vi "搜索变量函数.vi"(8 "错误输入":errorcluster caption="错误输入（无错误）", 11 "引用":refnum<k24>) -> (0 "错误输出":errorcluster, 1 "输出数组":string[](array[string]), 3 "引用输出":refnum<k24>)   [LabVIEW 2018]
uses:
  ScintillaNET.dll
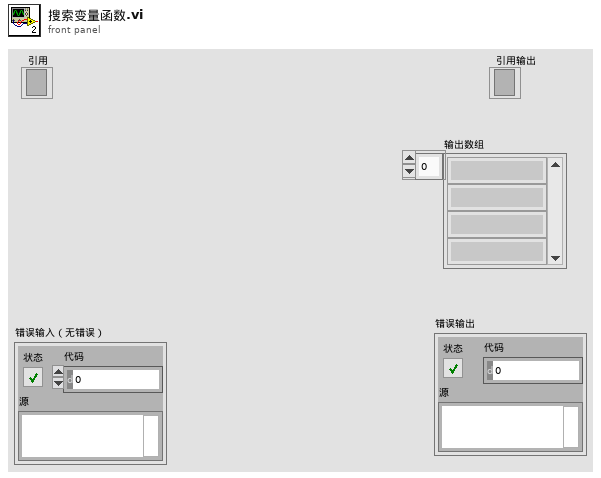
[diagram p1: front panel]
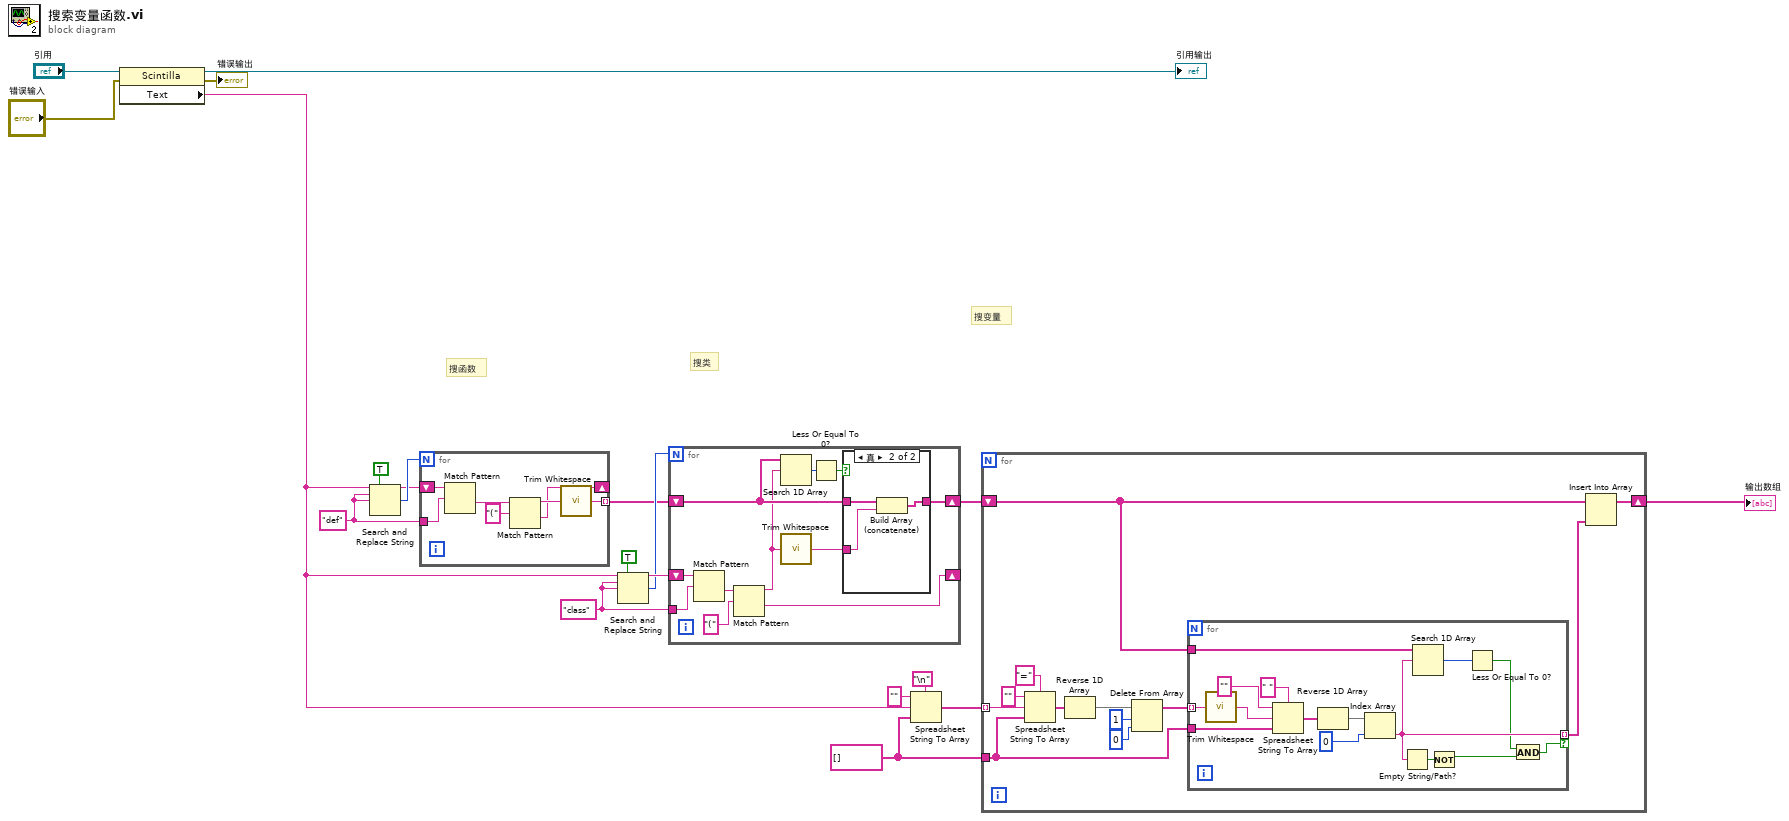
[diagram p0: block diagram]
diagram:
  w8 = string[] []
  w14 = "class" ("搜索字符串")
  w15 = "def" ("搜索字符串")
  # "搜变量"
  # "搜类"
  # "搜函数"
  n1 = property class="Scintilla"(reference="引用", error in="错误输入") -> (reference out=→"引用输出":refnum<k24>, error out=→"错误输出":errorcluster, "Text"=w4:string)
  n2 = Search and Replace String(replace all?=TRUE ("替换全部？(F)"), input string=w4, search string=w15, replace string=w15) -> (result string=w16:string, number of replacements=w17:i32)  [unwired: 4 in, 2 out]
  n3 = for {
    N: w17 -> [_]
    tunnel: [w23] -> w3 mode=indexing
    tunnel: w15 -> [w22]
    shift-right: [w21] -> _
    shift-left: w16 -> [w27]
    n4 = Match Pattern(string=w27, regular expression=w22) -> (after substring=w26:string)  [unwired: 1 in, 3 out]
    n5 = Match Pattern(string=w26, regular expression="(" ("正则表达式")) -> (before substring=w24:string, after substring=w21:string)  [unwired: 1 in, 2 out]
    n6 = call <vilib>:"Trim Whitespace.vi"("string"=w24) -> ("trimmed string"=w23:string)  [unwired: 1 in]
  }
  n7 = Search and Replace String(replace all?=TRUE ("替换全部？(F)"), input string=w4, search string=w14, replace string=w14) -> (result string=w13:string, number of replacements=w12:i32)  [unwired: 4 in, 2 out]
  n8 = for {
    N: w12 -> [_]
    tunnel: w14 -> [w35]
    shift-right: [w34] -> _
    shift-left: w13 -> [w38]
    shift-right: [w29] -> w2
    shift-left: w3 -> [w31]
    n9 = Match Pattern(string=w38, regular expression=w35) -> (after substring=w37:string)  [unwired: 1 in, 3 out]
    n10 = Match Pattern(string=w37, regular expression="(" ("正则表达式")) -> (before substring=w28:string, after substring=w34:string)  [unwired: 1 in, 2 out]
    n11 = Search 1D Array(1D array=w31, element=w28) -> (index of element=w33:i32)  [unwired: 1 in]
    n12 = call <vilib>:"Trim Whitespace.vi"("string"=w28) -> ("trimmed string"=w30:string)  [unwired: 1 in]
    n13 = Less Or Equal To 0?(x=w33) -> (x <= 0?=w32:bool)
    n14 = case shown="真" w32 {
      tunnel: w31 -> [w39 w42]
      tunnel: w30 -> [_ w41]
      tunnel: [w39 w40] -> w29
      frame False {
      }
      frame True {
        n15 = Build Array (concatenate)(w42, w41) -> (w40:string[])
      }
    }
  }
  n16 = Spreadsheet String To Array(delimiter (Tab)="\n", format string="" ("格式字符串"), spreadsheet string=w4, array type (2D Dbl)=w8) -> (array=w5:string[])
  n17 = for {
    tunnel: w5 -> [w47] mode=indexing
    tunnel: w8 -> [w46]
    shift-right: [w44] -> w1
    shift-left: w2 -> [w43]
    n18 = Spreadsheet String To Array(delimiter (Tab)="=" ("分隔符(Tab)"), format string="" ("格式字符串"), spreadsheet string=w47, array type (2D Dbl)=w46) -> (array=w51:string[])
    n19 = Reverse 1D Array(array=w51) -> (reversed array=w52:string[])
    n20 = Delete From Array(array=w52, length=1 ("长度"), index=0 ("索引")) -> (array with subset deleted=w48:string[])  [unwired: 1 out]
    n21 = for {
      tunnel: w48 -> [w69] mode=indexing
      tunnel: [w59] -> w45 mode=indexing if=w57
      tunnel: w46 -> [w62]
      tunnel: w43 -> [w60]
      n22 = call <vilib>:"Trim Whitespace.vi"("string"=w69) -> ("trimmed string"=w63:string)  [unwired: 1 in]
      n23 = Spreadsheet String To Array(delimiter (Tab)=" " ("分隔符(Tab)"), format string="" ("格式字符串"), spreadsheet string=w63, array type (2D Dbl)=w62) -> (array=w66:string[])
      n24 = Reverse 1D Array(array=w66) -> (reversed array=w65:string[])
      n25 = Index Array(array=w65, index=0 ("索引")) -> (element=w59:string)
      n26 = Empty String/Path?(string/path=w59) -> (empty?=w61:bool)
      n27 = Search 1D Array(1D array=w60, element=w59) -> (index of element=w58:i32)  [unwired: 1 in]
      n28 = Not(x=w61) -> (.not. x?=w55:bool)
      n29 = Less Or Equal To 0?(x=w58) -> (x <= 0?=w56:bool)
      n30 = And(x=w56, y=w55) -> (x .and. y?=w57:bool)
    }
    n31 = Insert Into Array(array=w43, new element=w45) -> (w44:string[])  [unwired: 1 in]
  }
  "输出数组" <- w1
